vi "Update.vi"(8 "error in (no error)":errorcluster, 11 "GroupLoggingControl in":refnum<class "GroupLoggingControl.lvclass">) -> (0 "error out":errorcluster, 3 "GroupLoggingControl out":refnum<class "GroupLoggingControl.lvclass">)   [LabVIEW 2020, in "VolatusGUIElements.lvlib" / "GroupLoggingControl.lvclass"]
uses:
  GroupLoggingControl.lvclass
  GroupLoggingControl.lvclass/GroupLoggingControl.ctl
  <vilib>/Utility/miscctls.llb/LVMapReplaceAction.ctl
  lv-vecto/Vecto/Channel DBL/Channel DBL.lvclass
  Volatus/VolatusAPI/VolatusAPI.lvclass
  <vilib>/httpClient/LabVIEWHTTPClient.lvlib
  VolatusGUI/GUI Element/GUI Element.lvclass
  C:/dev/lv20CE/relink/lv-volatus/VolatusGUI/GUI Element/GUI Element.lvclass
  C:/dev/lv20CE/relink/lv-volatus/VolatusGUIElements/GroupLoggingControl/GroupLoggingControl.lvclass
  C:/dev/lv20CE/relink/lv-volatus/VolatusGUI/OnValueChangeHandler/OnValueChangeHandler.lvclass
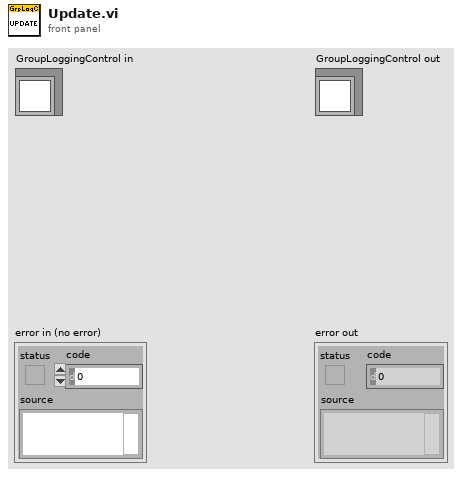
[diagram p1: front panel]
types:
  T1 = cluster{"Group":string, "Group Color":u32, "Button":bool}[]
  T2 = typedef "VolatusGUIElements.lvlib/GroupLoggingControl.lvclass/Target Info.ctl" = cluster{"Node":string, "Node Color":u32, "Groups":T3[]}
  T3 = typedef "VolatusGUIElements.lvlib/GroupLoggingControl.lvclass/Log Group.ctl" = cluster{"Status":T4, "Command Info":T5, "Logging":bool, "State":string}
  T4 = typedef "VolatusGUIElements.lvlib/GroupLoggingControl.lvclass/Log Group Status.ctl" = cluster{"Group":string, "Group Color":u32, "Button":bool}
  T5 = typedef "VolatusGUIElements.lvlib/GroupLoggingControl.lvclass/Command Info.ctl" = cluster{"Commanding":bool, "Cmd Time":dbl, "Group ID":string}
  T6 = typedef "LVMapReplaceAction.ctl" = enum32{"Modify Entry only if found", "Add or Modify Entry", "Delete Entry"}
  T7 = cluster{"State":string, "Log":string, "Groups":cluster{"Group":string, "State":string}[]}
  T8 = cluster{"Group":string, "Group Color":u32, "Button":bool}
  T9 = cluster{"Node":string, u32, cluster{"Group":string, "Group Color":u32, "Button":bool}[]}
  T10 = cluster{string, string, cluster{"Node":string, u32, cluster{"Group":string, "Group Color":u32, "Button":bool}[]}[], "Groups":cluster{"Group":string, "Group Color":u32, "Button":bool}[]}
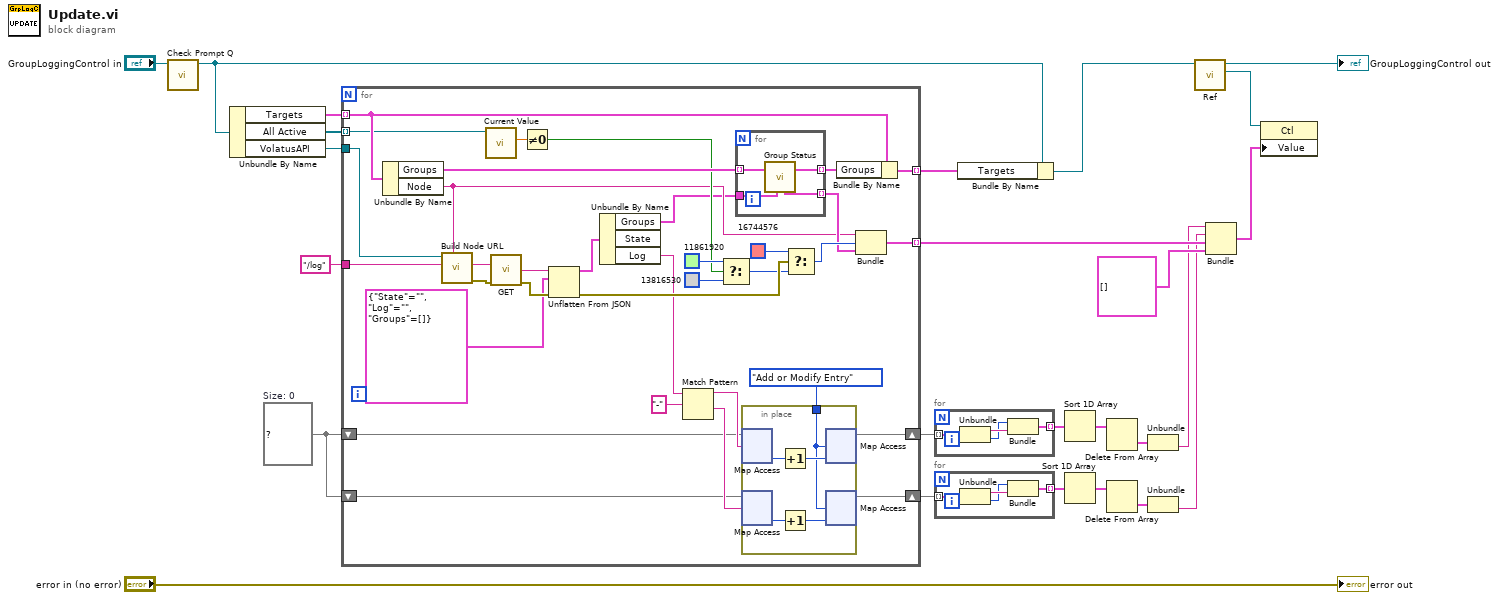
[diagram p0: block diagram]
diagram:
  w18 = map{string, i32} {}  # Size: 0
  n1 = call "Check Prompt Q.vi"("LoggingControl in"="GroupLoggingControl in") -> ("LoggingControl out"=w20:refnum<class "GroupLoggingControl.lvclass">)  [unwired: 9 in, 1 out]
  n2 = Unbundle By Name(w20) -> ("Targets"=w24:T2[], "All Active"=w19:refnum<class "Channel DBL.lvclass">[], "VolatusAPI"=w17:refnum<class "VolatusAPI.lvclass">)
  n3 = for {
    tunnel: w24 -> [w50] mode=indexing
    tunnel: [w53] -> w23 mode=indexing
    tunnel: [w48] -> w14 mode=indexing
    tunnel: w19 -> [w46] mode=indexing
    shift-right: [w29] -> w7
    shift-left: w18 -> [w28]
    shift-right: [w30] -> w6
    shift-left: w18 -> [w27]
    tunnel: w17 -> [w39]
    tunnel: "/log" -> [w37]
    n4 = Unbundle By Name(w50) -> ("Groups"=w52:T3[], "Node"=w38:string)
    n5 = call "Build Node URL.vi"("Node Name"=w38, "Path"=w37, "VolatusAPI in"=w39) -> ("error out"=w44:errorcluster, "Request URL"=w42:string)  [unwired: 6 in, 1 out]
    n6 = call "Current Value.vi"("Channel in"=w46) -> ("Scaled"=w47:dbl)  [unwired: 6 in, 4 out]
    n7 = call <vilib>:"GET.vi"("url"=w42, "error in (no error)"=w44) -> ("body"=w43:string, "error out"=w41:errorcluster)  [unwired: 10 in, 2 out]
    n8 = Not Equal To 0?(x=w47) -> (x != 0?=w45:bool)
    n9 = Unflatten From JSON(JSON string=w43, type and defaults=T7 {"State"="", "Log"="", "Groups"=[]} ("output cluster"), error in (no error)=w41) -> (value=w32:T7, error out=w59:errorcluster)  [unwired: 4 in]
    n10 = Unbundle By Name(w32) -> ("Groups"=w26:cluster{"Group":string, "State":string}[], "Log"=w31:string)  [unwired: 1 out]
    n11 = Match Pattern(string=w31, regular expression="-") -> (before substring=w34:string, after substring=w33:string)  [unwired: 1 in, 2 out]
    n12 = Select(t=u32 11861920, s=w45, f=u32 13816530) -> (s? t:f=w56:u32)
    n13 = for {
      tunnel: w52 -> [w68] mode=indexing
      tunnel: [w67] -> w51 mode=indexing
      tunnel: [w66] -> w49 mode=indexing
      tunnel: w26 -> [w65]
      n14 = call "Group Status.vi"("Log Group"=w68, "Groups"=w65) -> ("Group Status"=w67:T8, "Group"=w66:T3)  [unwired: 4 in]
    }
    n15 = in-place {
      in-place-border: LVMapReplaceAction."Add or Modify Entry" ("action") -> [w60]
      n16 = in-place-map #1(w28, w34) -> (w64:i32)  [unwired: 1 in, 1 out]
      n17 = in-place-map #2(w27, w33) -> (w63:i32)  [unwired: 1 in, 1 out]
      n18 = Increment(x=w64) -> (x+1=w61:i32)
      n19 = Increment(x=w63) -> (x+1=w62:i32)
      n20 = in-place-map #1(w61, w60) -> (w29:map{string, i32})  [unwired: 2 out]
      n21 = in-place-map #2(w62, w60) -> (w30:map{string, i32})  [unwired: 2 out]
    }
    n22 = Select(t=u32 16744576, s=w59, f=w56) -> (s? t:f=w54:u32)
    n23 = Bundle By Name(cluster=w50, "Groups"=w49) -> (w48:T2)
    n24 = Bundle("Node"=w38, w54, w51) -> (w53:T9)  [unwired: 1 in]
  }
  n25 = for {
    tunnel: w7 -> [w72] mode=indexing
    tunnel: [w69] -> w13 mode=indexing
    n26 = Unbundle(w72) -> (w71:string, w70:i32)
    n27 = Bundle(w70, w71) -> (w69:cluster{i32, string})  [unwired: 1 in]
  }
  n28 = for {
    tunnel: w6 -> [w76] mode=indexing
    tunnel: [w73] -> w8 mode=indexing
    n29 = Unbundle(w76) -> (w75:string, w74:i32)
    n30 = Bundle(w74, w75) -> (w73:cluster{i32, string})  [unwired: 1 in]
  }
  n31 = Bundle By Name(cluster=w20, "Targets"=w14) -> (w15:refnum<class "GroupLoggingControl.lvclass">)
  n32 = Sort 1D Array(array=w13) -> (sorted array=w12:cluster{i32, string}[])
  n33 = Sort 1D Array(array=w8) -> (sorted array=w9:cluster{i32, string}[])
  n34 = Delete From Array(array=w12) -> (deleted portion=w11:cluster{i32, string})  [unwired: 2 in, 1 out]
  n35 = Delete From Array(array=w9) -> (deleted portion=w10:cluster{i32, string})  [unwired: 2 in, 1 out]
  n36 = Unbundle(w11) -> (w5:string)  [unwired: 1 out]
  n37 = Unbundle(w10) -> (w4:string)  [unwired: 1 out]
  n38 = call "Ref.vi"("GUI Element in"=w15) -> ("Ref"=w2:refnum<vi>, "GUI Element out"=→"GroupLoggingControl out":refnum<class "GroupLoggingControl.lvclass">)  [unwired: 9 in]
  n39 = Bundle(w5, w4, w23, "Groups"=T1 []) -> (w1:T10)  [unwired: 1 in]
  n40 = property class="Ctl"(reference=w2, "Value"=w1) -> ()  [unwired: 1 in, 2 out]
  "error out" <- "error in (no error)"
